vi "Init.vi"(8 "error in (no error)":errorcluster, 9 "Clock type":enum8{"Internal", "External", "PXI"}(ring), 10 "Slot":u16) -> (0 "error out":errorcluster, 3 "MagiQmw3 out":refnum<class "MagiQmw3.lvclass">)   [LabVIEW 2012, in "MagiQmw3.lvclass"]
uses:
  MagiQmw3.lvclass
  MagiQmw3.lvclass/MagiQmw3.ctl
panel:
  out "Clock ok":bool
  out "Ref dividers ok":bool[](array[boolean])
  out "path":path
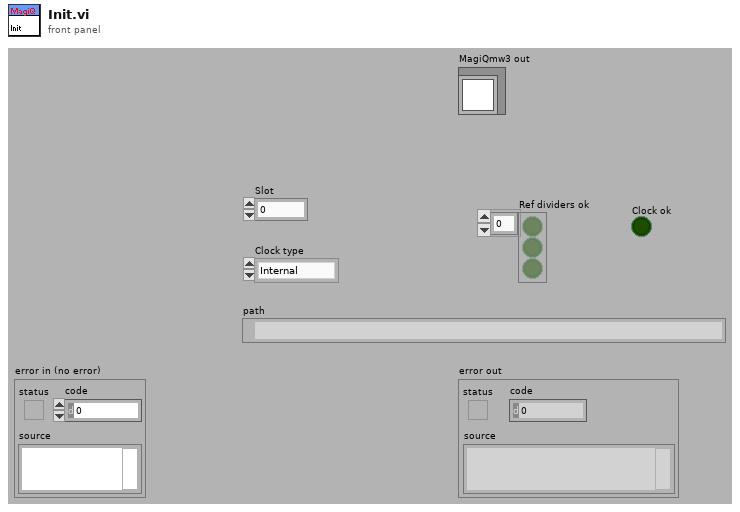
[diagram p1: front panel]
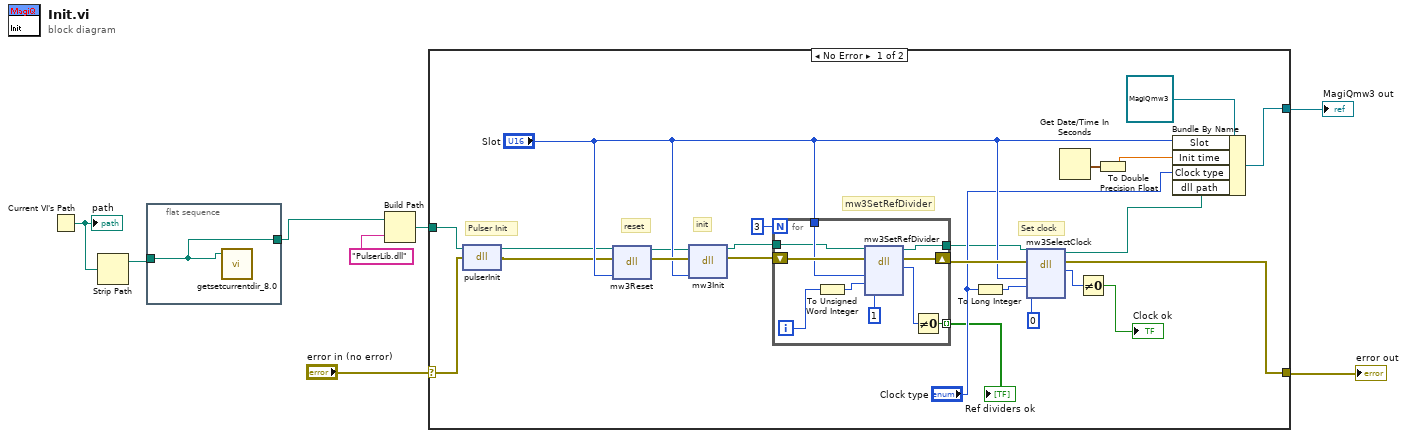
[diagram p0: block diagram]
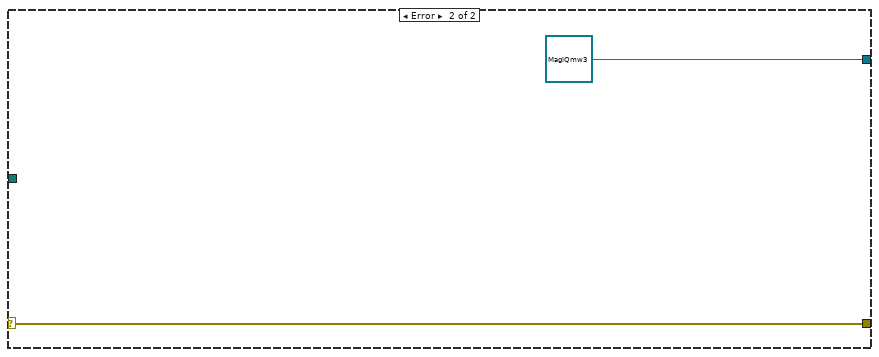
[diagram p2: hidden frame]
diagram:
  n1 = Current VI's Path() -> (path=w3:path)
  "path" <- w3
  n2 = Strip Path(path=w3) -> (stripped path=w2:path)  [unwired: 1 out]
  n3 = flat-sequence {
    tunnel: w2 -> [w9]
    tunnel: [w9] -> w1
    frame #0 {
      n4 = call "getsetcurrentdir_8.0.vi"("Set Directory"=w9) -> ()  [unwired: 5 in]
    }
  }
  n5 = Build Path(base path=w1, name or relative path="PulserLib.dll") -> (appended path=w4:path)
  n6 = case shown="No Error" "error in (no error)" {
    selector: "error in (no error)" -> [w14 w45]
    tunnel: [w24 w45] -> w7
    tunnel: [w33 refnum<class "MagiQmw3.lvclass"> refnum ("MagiQmw3 in")] -> w6
    tunnel: w4 -> [w16 _]
    frame No Error {
      # "Pulser Init"
      # "Set clock"
      # "mw3SetRefDivider"
      # "reset"
      # "init"
      n7 = dll-call lib="C:/Documents and Settings/Administrator/My Documents/VIs/magiq/PulserLib.dll" fn="pulserInit"(path in=w16, error in=w14) -> (path out=w15:path, error out=w13:errorcluster)  [unwired: 2 in]
      n8 = dll-call lib="PulserLib.dll" fn="mw3Reset"(path in=w15, error in=w13, "slot"="Slot") -> (path out=w20:path, error out=w29:errorcluster)  [unwired: 3 in]
      n9 = dll-call lib="PulserLib.dll" fn="mw3Init"(path in=w20, error in=w29, "slot"="Slot") -> (path out=w19:path, error out=w27:errorcluster)  [unwired: 3 in]
      n10 = for {
        N: 3 -> [_]
        shift-right: [w43] -> w26
        shift-left: w27 -> [w41]
        tunnel: "Slot" -> [w38]
        tunnel: w19 -> [w37]
        tunnel: [w36] -> w18
        tunnel: [w34] -> w12 mode=indexing
        i -> [w39]
        n11 = To Unsigned Word Integer(number=w39) -> (unsigned 16bit integer=w40:u16)
        n12 = dll-call lib="PulserLib.dll" fn="mw3SetRefDivider"(path in=w37, error in=w41, "slot"=w38, "ch"=w40, "val"=u64 1) -> (path out=w36:path, error out=w43:errorcluster, "return type"=w35:i32)  [unwired: 4 in]
        n13 = Not Equal To 0?(x=w35) -> (x != 0?=w34:bool)
      }
      "Ref dividers ok" <- w12
      n14 = To Long Integer(number="Clock type") -> (32bit integer=w23:i32)
      n15 = dll-call lib="PulserLib.dll" fn="mw3SelectClock"(path in=w18, error in=w26, "slot"="Slot", "clockType"=w23, "clkMhz"=u64 0) -> (path out=w17:path, error out=w24:errorcluster, "return type"=w11:i32)  [unwired: 4 in]
      n16 = Get Date/Time In Seconds() -> (seconds since 1Jan1904=w32:timestamp)
      n17 = Not Equal To 0?(x=w11) -> (x != 0?=→"Clock ok":bool)
      n18 = To Double Precision Float(number=w32) -> (double precision float=w31:dbl)
      n19 = Bundle By Name(cluster=refnum<class "MagiQmw3.lvclass"> refnum ("MagiQmw3 in"), "Slot"="Slot", "Init time"=w31, "Clock type"="Clock type", "dll path"=w17) -> (w33:refnum<class "MagiQmw3.lvclass">)
    }
    frame Error {
    }
  }
  "error out" <- w7
  "MagiQmw3 out" <- w6
